vi "NIIE_Magic Active Layer Constant.vi"() -> (3 "Magic Constant":i32=-99)   [LabVIEW 2021]
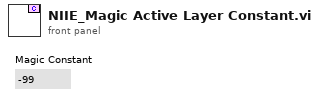
[diagram p1: front panel]
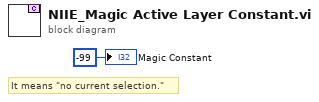
[diagram p0: block diagram]
diagram:
  # "It means \"no current selection.\""
  "Magic Constant" <- -99 ("#Active Layer")
